vi "Stop and Stop on Error.vi"(7 "Action":enum16{"Check", "Reset"}(ring)=enum."Reset", 8 "error in (no error)":errorcluster, 10 "Stop":bool) -> (0 "error out":errorcluster, 2 "Stop?":bool)   [LabVIEW 2016, in "Shared Variable Interface.lvlib"]
uses:
  Shared Variable Interface.lvlib
  <vilib>/ErrorRing/Error Ring.xnode
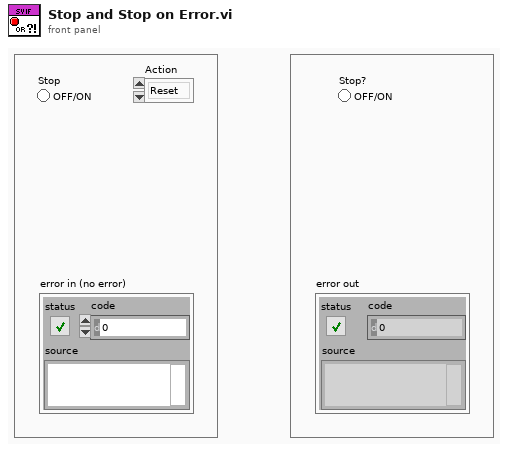
[diagram p1: front panel]
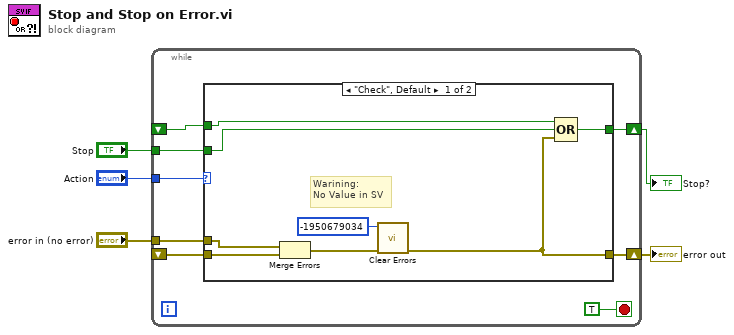
[diagram p0: block diagram]
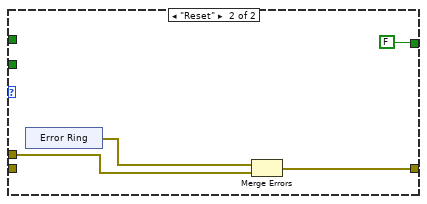
[diagram p2: hidden frame]
diagram:
  n1 = while {
    tunnel: "Action" -> [w13]
    tunnel: "error in (no error)" -> [w11]
    shift-right: [w10] -> w3
    shift-left: _ -> [w9]
    shift-right: [w8] -> w1
    shift-left: _ -> [w7]
    tunnel: "Stop" -> [w6]
    stop <- TRUE stop-if-true
    n2 = case shown="\"Check\", Default" w13 {
      tunnel: w11 -> [w21 w24]
      tunnel: [w15 w25] -> w10
      tunnel: w9 -> [w20 _]
      tunnel: [w17 FALSE] -> w8
      tunnel: w7 -> [w19 _]
      tunnel: w6 -> [w18 _]
      frame "Check", Default {
        # "Warining:\nNo Value in SV"
        n3 = Merge Errors(w21, w20) -> (w16:errorcluster)
        n4 = call <vilib>:"Clear Errors.vi"("error in (no error)"=w16, "specific error code to clear (0: all)"=-1950679034) -> ("error out"=w15:errorcluster)  [unwired: 4 in, 1 out]
        n5 = Compound Arithmetic op=OR(w19, w18, w15) -> (w17:bool)
      }
      frame "Reset" {
        n6 = xnode "Error Ring"() -> ("error out"=w23:errorcluster)
        n7 = Merge Errors(w23, w24) -> (w25:errorcluster)
      }
    }
  }
  "error out" <- w3
  "Stop?" <- w1
